vi "testInvParam.vi"() -> ()   [LabVIEW 2014]
uses:
  ICRMKinematics.llb/nloptIKParams.ctl
  ICRMKinematics.llb/jntLims.ctl
  <vilib>/Analysis/Matrix/Datatypes/RealMatrix.ctl
  ICRMKinematics.llb/knPms11A.ctl
  <vilib>/Analysis/Matrix/NI_Matrix.lvlib
panel:
  in  "knPM":T1={"tx01"=20.0, "ty01"=20.0, "tz01"=20.0, "ry01"=0.2, "rz01"=0.2, "tx23"=1.0, "ry34"=0.2, "rz34"=0.2, "cathL"=10.0, "ry45"=0.2, "rz45"=0.2}
  in  "kn0":T1={"tx01"=806.0, "ty01"=-66.0, "tz01"=-28.0, "ry01"=0.0, "rz01"=-0.24, "tx23"=8.2, "ry34"=0.0, "rz34"=0.0, "cathL"=98.0, "ry45"=0.0, "rz45"=0.0}
  out "kn":T1={"tx01"=820.8148148148148, "ty01"=-59.58024691358025, "tz01"=-28.0, "ry01"=0.0, "rz01"=-0.2696296296296296, "tx23"=8.05185185185185, "ry34"=0.19259259259259257, "rz34"=-0.14814814814814814, "cathL"=97.25925925925925, "ry45"=0.0, "rz45"=-0.02962962962962963}
  out "retCodeOut":i32(ring)=5 items=["forced stop"=-5, "roundoff limited"=-4, "out of memory"=-3, "invalid args"=-2, "general failure"=-1, "zero"=0, "success"=1, "error below errTol"=2, "function step tol reached"=3, "x step tol reached"=4, "max fun evals"=5, "max time"=6]
  out "fmin":dbl=176352.04291218042
  out "error out":errorcluster
  out "qps0":dbl[](array[numeric])=[0.2666666666666666, -0.13333333333333333, 0.04444444444444447, -0.13333333333333333, -9.62962962962963]
  in  "qp0":dbl[](array[numeric])=[0.0, 0.0, 0.0, 0.0, 0.0]
  in  "data":T3(array[cluster])=array[15004 elements]
  in  "q0Lims":T4={"dn"=[-0.4, -0.2, -0.2, -0.2, -10.0], "up"=[0.4, 0.2, 0.2, 0.2, 10.0]}
  in  "nlParams":T5={"maxIts"=1000.0, "maxTimeSec"=60.0, "nlMethod"=enum."GN_DIRECT", "errTol"=1e-06, "tolFun"=1e-06, "tolX"=1e-06}
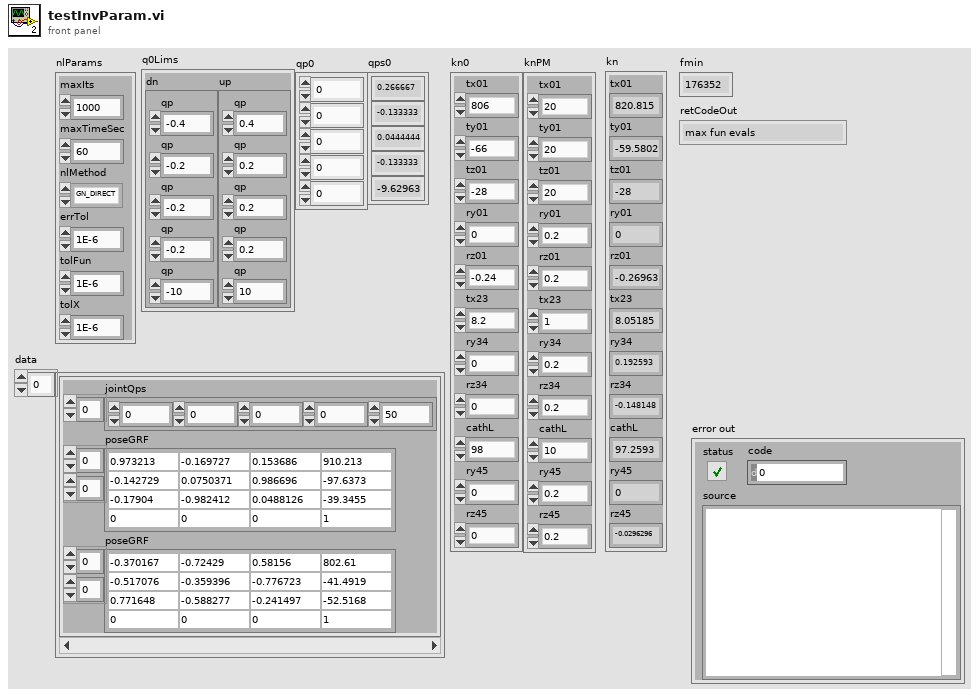
[diagram p1: front panel]
types:
  T1 = typedef "knPms11A.ctl" = cluster{"tx01":dbl, "ty01":dbl, "tz01":dbl, "ry01":dbl, "rz01":dbl, "tx23":dbl, "ry34":dbl, "rz34":dbl, "cathL":dbl, "ry45":dbl, "rz45":dbl}
  T2 = typedef "NI_Matrix.lvlib/RealMatrix.ctl" = dbl[][]
  T3 = cluster{"jointQps":dbl[], "poseGRF":T2, "poseGRF":T2}[]
  T4 = typedef "jntLims.ctl" = cluster{"dn":dbl[], "up":dbl[]}
  T5 = typedef "nloptIKParams.ctl" = cluster{"maxIts":dbl, "maxTimeSec":dbl, "nlMethod":enum16{"GN_DIRECT", "GN_DIRECT_L", "GN_DIRECT_L_NOSCAL", "GN_DIRECT_L_RAND", "GN_DIRECT_L_RAND_NOSCAL", "GN_DIRECT_NOSCAL", "GN_ESCH", "GN_ISRES", "GN_MLSL", "GN_MLSL_LDS", "GN_ORIG_DIRECT", "GN_ORIG_DIRECT_L", "LN_BOBYQA", "LN_COBYLA", "LN_NELDERMEAD", "LN_NEWUOA", "LN_NEWUOA_BOUND", "LN_PRAXIS", "LN_SBPLX"}, "errTol":dbl, "tolFun":dbl, "tolX":dbl}
  T6 = cluster{"nlParams":T5, "qp0":dbl[], "q0dn":dbl[], "q0up":dbl[], "kn0":T1, "knPM":T1}
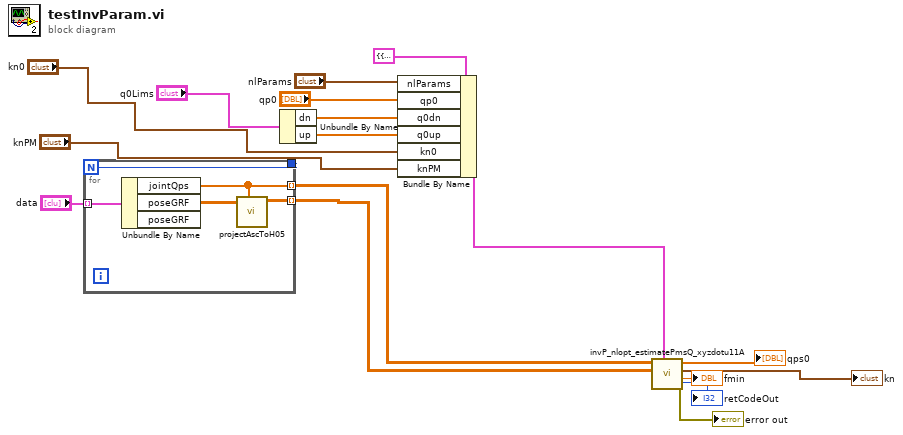
[diagram p0: block diagram]
diagram:
  n1 = for {
    N -> [w21]
    tunnel: "data" -> [w22] mode=indexing
    tunnel: [w19] -> w11 mode=indexing
    tunnel: [w21] -> _
    tunnel: [w18] -> w10 mode=indexing
    n2 = Unbundle By Name(w22) -> ("jointQps"=w19:dbl[], "poseGRF"=w20:T2)  [unwired: 1 out]
    n3 = call "projectAscToH05.vi"("qps"=w19, "ascGRF"=w20) -> ("ascH05"=w18:T2)  [unwired: 9 in]
  }
  n4 = Unbundle By Name("q0Lims") -> ("dn"=w13:dbl[], "up"=w12:dbl[])
  n5 = Bundle By Name(cluster=T6 {"nlParams"={"maxIts"=100000.0, "maxTimeSec"=60.0, "nlMethod"=enum."GN_DIRECT", "errTol"=1e-06, "tolFun"=1e-06, "tolX"=1e-06}, "qp0"=[0.0, 0.0, 0.0, 0.0, 0.0], "q0dn"=[-0.4, -0.2, -0.2, -0.2, -10.0], "q0up"=[0.4, 0.2, 0.2, 0.2, 10.0], "kn0"={"tx01"=806.0, "ty01"=-66.0, "tz01"=-28.0, "ry01"=0.0, "rz01"=-0.24, "tx23"=8.2, "ry34"=0.0, "rz34"=0.0, "cathL"=98.0, "ry45"=0.0, "rz45"=0.0}, "knPM"={"tx01"=20.0, "ty01"=20.0, "tz01"=20.0, "ry01"=0.2, "rz01"=0.2, "tx23"=1.0, "ry34"=0.2, "rz34"=0.2, "cathL"=10.0, "ry45"=0.2, "rz45"=0.2}} ("in"), "nlParams"="nlParams", "qp0"="qp0", "q0dn"=w13, "q0up"=w12, "kn0"="kn0", "knPM"="knPM") -> (w2:T6)
  n6 = call "invP_nlopt_estimatePmsQ_xyzdotu11A.vi"("in"=w2, "ascH05"=w10, "jointQps"=w11) -> ("error out"=→"error out":errorcluster, "fmin"=→"fmin":dbl, "kn"=→"kn":T1, "qps0out"=→"qps0":dbl[], "retCodeOut"=→"retCodeOut":i32)  [unwired: 4 in]
